vi "Read Heigth.vi"(11 "Rectangle in":refnum<class "Rectangle.lvclass">) -> (2 "Heigth":dbl, 3 "Rectangle out":refnum<class "Rectangle.lvclass">)   [LabVIEW 2018, in "Rectangle.lvclass"]
uses:
  Rectangle.lvclass
  Rectangle.lvclass/Rectangle.ctl
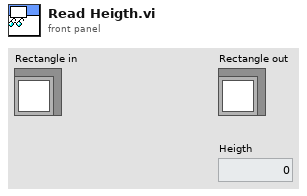
[diagram p1: front panel]
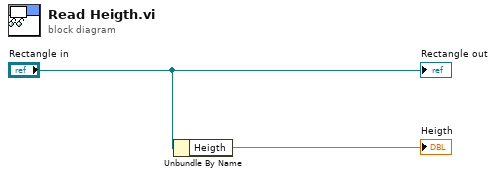
[diagram p0: block diagram]
diagram:
  n1 = Unbundle By Name("Rectangle in") -> ("Heigth"=→"Heigth":dbl)
  "Rectangle out" <- "Rectangle in"
